vi "全局变量.vi"() -> ()   [LabVIEW 2018]
panel:
  out "字符串":string
  in  "数值":dbl
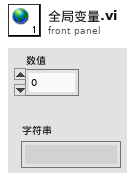
[diagram p1: front panel]
diagram:
